vi "ReadTemperatures.vi"(8 "Error In":errorcluster, 11 "Temperature Task In":refnum<k21>) -> (0 "Error Out":errorcluster, 2 "Raw Data":dbl[][](array[numeric]), 3 "Temperature Task Out":refnum<k21>)   [LabVIEW 2012]
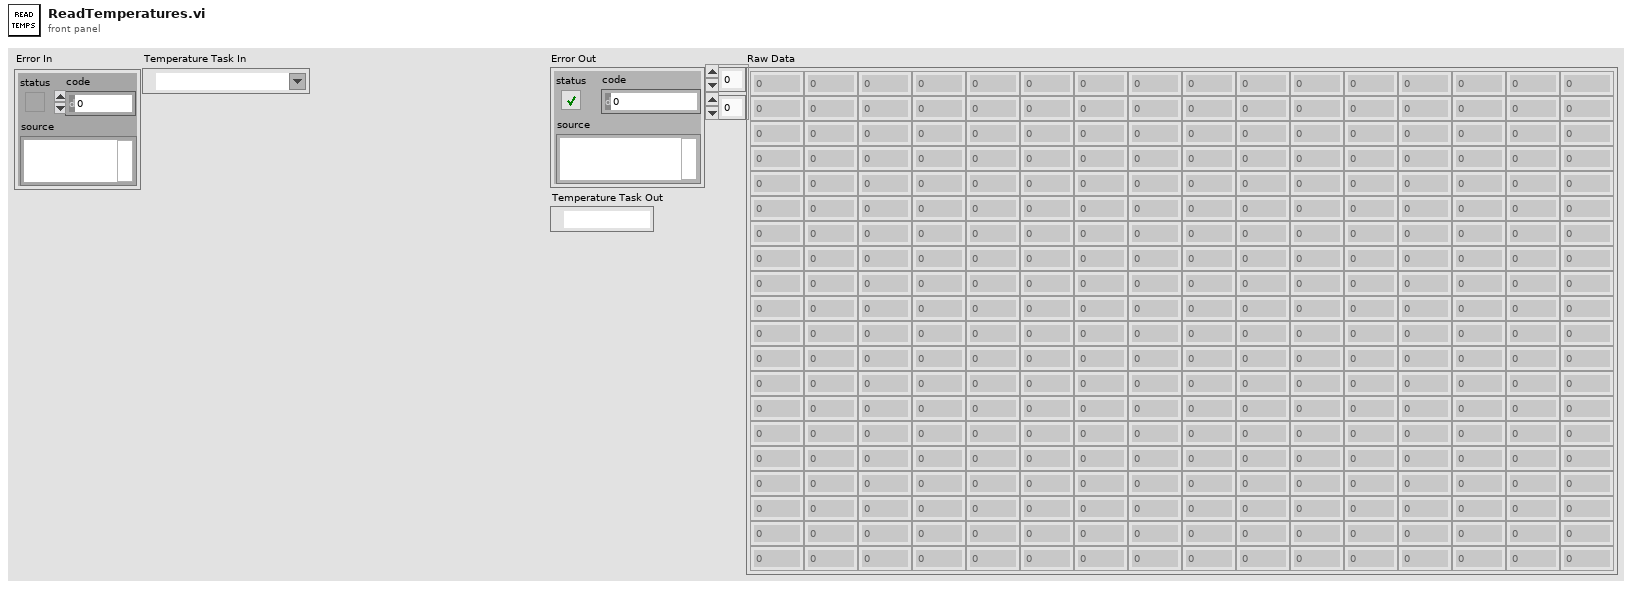
[diagram p1: front panel]
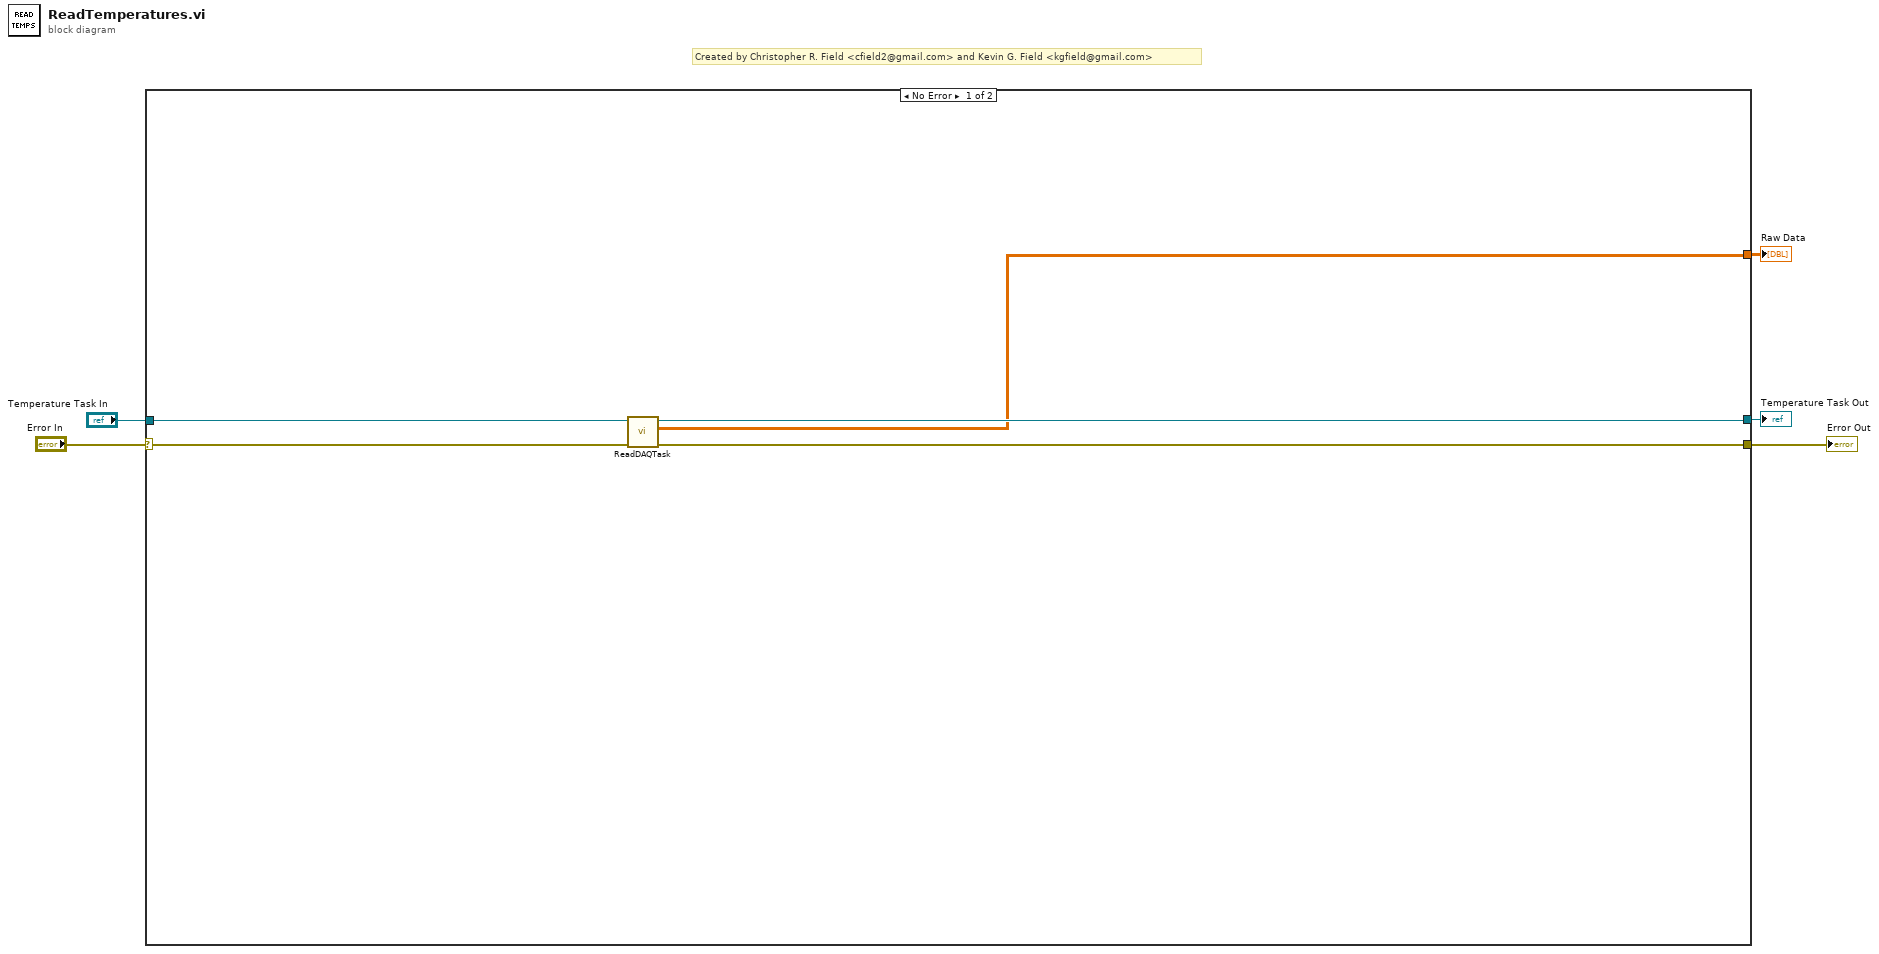
[diagram p0: block diagram]
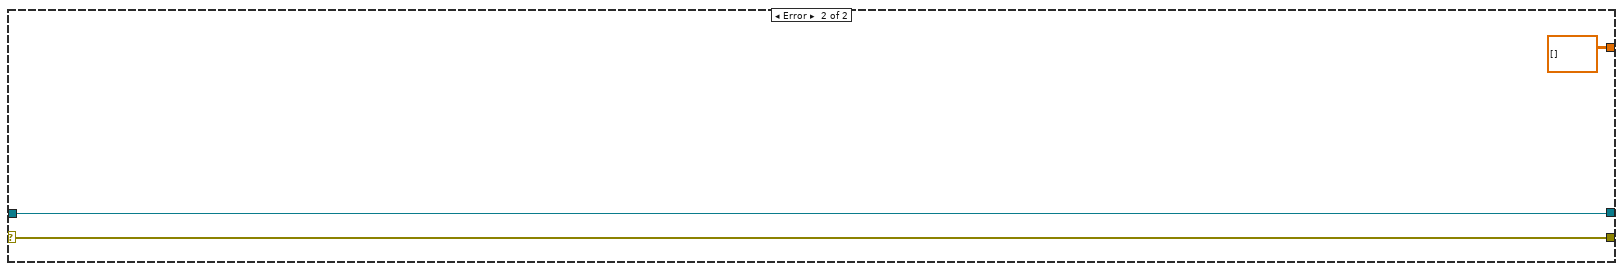
[diagram p2: hidden frame]
diagram:
  # "Created by Christopher R. Field <cfield2@gmail.com> and Kevin G. Field <kgfield@gmail.com>"
  n1 = case shown="No Error" "Error In" {
    selector: "Error In" -> [w9 w12]
    tunnel: "Temperature Task In" -> [w10 w13]
    tunnel: [w8 w13] -> w2
    tunnel: [w7 w12] -> w3
    tunnel: [w6 dbl[][] [] ("Data")] -> w1
    frame No Error {
      n2 = call "ReadDAQTask.vi"("Error In"=w9, "DAQ Task In"=w10) -> ("Error Out"=w7:errorcluster, "Data"=w6:dbl[][], "DAQ Task Out"=w8:refnum<k21>)  [unwired: 7 in]
    }
    frame Error {
    }
  }
  "Error Out" <- w3
  "Temperature Task Out" <- w2
  "Raw Data" <- w1
